vi "terminate.vi"(8 "error in (no error)":errorcluster, 11 "Stimulator090724 in":refnum<class "Stimulator090724Scaffold.lvclass">) -> (0 "error out":errorcluster, 3 "Stimulator090724 out":refnum<class "Stimulator090724Scaffold.lvclass">)   [LabVIEW 2010, in "Stimulator090724Scaffold.lvclass"]
doc: "The dynamic dispatch version of this VI terminates the plug-in object by releasing all of its resources."
uses:
  Stimulator090724Scaffold.lvclass
  Stimulator090724Scaffold.lvclass/Stimulator090724Scaffold.ctl
  Clock/GenericClock/GenericClock/GenericClock.lvclass
  GenericStimulator/GenericStimulator/GenericStimulator.lvclass
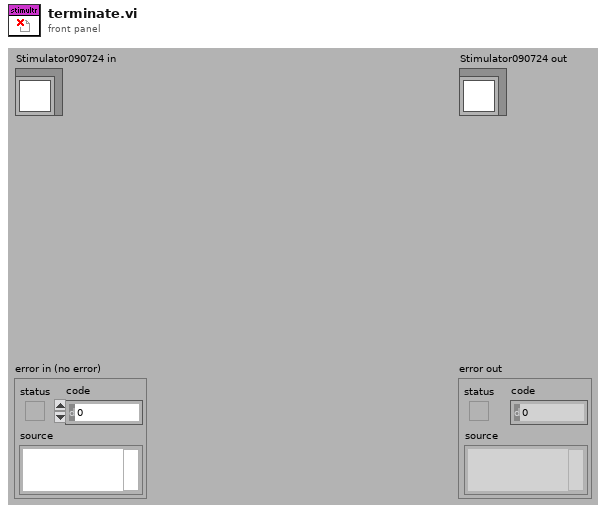
[diagram p1: front panel]
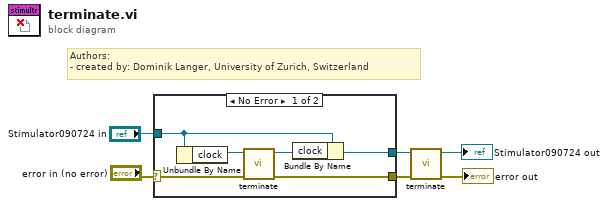
[diagram p0: block diagram]
diagram:
  # "Authors: \n- created by: Dominik Langer, University of Zurich, Switzerland"
  n1 = case shown="No Error" "error in (no error)" {
    selector: "error in (no error)" -> [w12 w13]
    tunnel: [w9 w13] -> w5
    tunnel: "Stimulator090724 in" -> [w10 w14]
    tunnel: [w8 w14] -> w4
    frame No Error {
      n2 = Unbundle By Name(w10) -> ("clock"=w11:refnum<class "GenericClock.lvclass">)
      n3 = call-dynamic "terminate.vi"("error in (no error)"=w12, "GenericPlugin in"=w11) -> ("error out"=w9:errorcluster, "GenericPlugin out"=w7:refnum<class "GenericClock.lvclass">)  [unwired: 8 out]
      n4 = Bundle By Name(cluster=w10, "clock"=w7) -> (w8:refnum<class "Stimulator090724Scaffold.lvclass">)
    }
    frame Error {
    }
  }
  n5 = call-parent "terminate.vi"("error in (no error)"=w5, "GenericPlugin in"=w4) -> ("error out"=→"error out":errorcluster, "GenericPlugin out"=→"Stimulator090724 out":refnum<class "Stimulator090724Scaffold.lvclass">)  [unwired: 8 out]
